vi "traffic light.vi"() -> ()   [LabVIEW 2011]
panel:
  in  "stop 2":bool
  out "stop":bool
  out "go":bool
  out "ready":bool
  in  "Green":bool
  in  "Yellow":bool
  in  "Red":bool
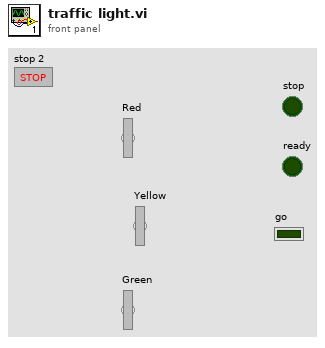
[diagram p1: front panel]
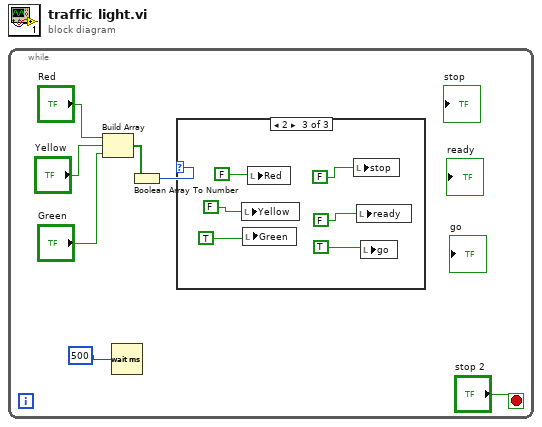
[diagram p0: block diagram]
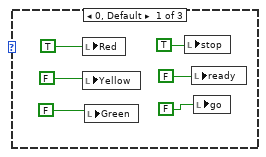
[diagram p2: hidden frame]
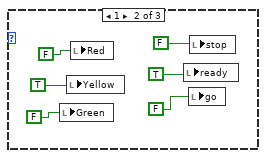
[diagram p3: hidden frame]
diagram:
  n1 = while {
    stop <- "stop 2" stop-if-true
    n2 = Build Array("Red", "Yellow", "Green") -> (w4:bool[])
    n3 = Wait (ms)(milliseconds to wait=500) -> ()  [unwired: 1 out]
    n4 = Boolean Array To Number(Boolean array=w4) -> (number=w3:u32)
    n5 = case shown="2" w3 {
      frame 0, Default {
        n6 = local write "Red"(TRUE) -> ()
        n7 = local write "Yellow"(FALSE) -> ()
        n8 = local write "Green"(FALSE) -> ()
        n9 = local write "stop"(TRUE) -> ()
        n10 = local write "ready"(FALSE) -> ()
        n11 = local write "go"(FALSE) -> ()
      }
      frame 1 {
        n12 = local write "Green"(FALSE) -> ()
        n13 = local write "Yellow"(TRUE) -> ()
        n14 = local write "Red"(FALSE) -> ()
        n15 = local write "ready"(TRUE) -> ()
        n16 = local write "go"(FALSE) -> ()
        n17 = local write "stop"(FALSE) -> ()
      }
      frame 2 {
        n18 = local write "Yellow"(FALSE) -> ()
        n19 = local write "Green"(TRUE) -> ()
        n20 = local write "Red"(FALSE) -> ()
        n21 = local write "stop"(FALSE) -> ()
        n22 = local write "ready"(FALSE) -> ()
        n23 = local write "go"(TRUE) -> ()
      }
    }
  }
